vi "SERIAL_StreamProcessor.vi"() -> ()   [LabVIEW 2014, in "navX-MXP IMU.lvlib"]
uses:
  navX-MXP IMU.lvlib
  COMMON/TypeDefs/navX Device TypeDef.ctl
  COMMON/TypeDefs/Value TypeDefs/navX Interface Protocol.ctl
  <vilib>/Rock Robotics/WPI/SPI/WPI_SPIDevRef.ctl
  <vilib>/Rock Robotics/SystemInterfaces/Typedef/FPGA_TypedefDigitalModule.ctl
  <vilib>/Rock Robotics/SystemInterfaces/spilib/spi_bus.ctl
  <vilib>/Rock Robotics/WPI/I2C/WPI_I2CDevRef.ctl
  <vilib>/Rock Robotics/SystemInterfaces/i2clib/i2c_bus.ctl
  <vilib>/Rock Robotics/WPI/SerialPort/WPI_SerialPortRef.ctl
  COMMON/TypeDefs/Data TypeDefs/navX Board Information.ctl
  COMMON/TypeDefs/Value TypeDefs/navX NAVX_BOARD_CAPABILITY.ctl
  COMMON/TypeDefs/Value TypeDefs/navX NAVX_BOARD_YAW_AXIS.ctl
  COMMON/TypeDefs/Data TypeDefs/navX Status Data.ctl
  COMMON/TypeDefs/Value TypeDefs/navX NAVX_OP_STATUS.ctl
  COMMON/TypeDefs/Value TypeDefs/navX NAVX_CAL_STATUS.ctl
  COMMON/TypeDefs/Value TypeDefs/navX NAVX_SELFTEST_STATUS.ctl
  COMMON/TypeDefs/Value TypeDefs/navX NAVX_SENSOR_STATUS.ctl
  COMMON/TypeDefs/Data TypeDefs/navX Offsets Data.ctl
  COMMON/TypeDefs/Value TypeDefs/navX Update Rate.ctl
  COMMON/TypeDefs/Value TypeDefs/navX Serial Mode.ctl
  <vilib>/Platform/TimedLoop/XDataNode/timing_clust.ctl
  <vilib>/Platform/TimedLoop/XDataNode/nitl_modes.ctl
  <vilib>/Platform/TimedLoop/XDataNode/wakeup.ctl
  COMMON/TypeDefs/Value TypeDefs/navX Device Registers.ctl
  <vilib>/Rock Robotics/SystemInterfaces/Utilities/FPGA_UtilitiesRead LocalTime.vi
  <vilib>/platform/TimedLoop/XDataNode/XDataNode.xnode
  <vilib>/Platform/TimedLoop/XDataNode/XDNodeRunTimeDep.lvlib
  NI WPI/NI WPI Serial USB.lvlib
panel:
  in  "navX DevRef":T1={"navX Interface Protocol"=enum."SPI", "navX Interface Protocol TypeDefs"={"SPIDevRef"={"DevStatus"={"status"=FALSE, "code"=0, "source"=""}, "Handle"=0, "Controller"=enum."Controller 1", "SPI Bus"=enum."SPI On-Board, CS0"}, "I2CDevRef"={"DevStatus"={"status"=FALSE, "code"=0, "source"=""}, "Controller"=enum."Controller 1", "Device Address"=0, "Handle"=0, "I2C Bus"=enum."Invalid"}, "SerialPortRef"={"DevStatus"={"status"=FALSE, "code"=0, "source"=""}, "Serial Port Name"=""}}, "navX System Information"={"Board Information"={"WhoAmI (50 | 0x32)"=0, "Board Revision"=0, "Firmware Major Version"=0, "Firmware Minor Version"=0, "NAVX_BOARD_CAPABILITY"={"OMNIMOUNT"=FALSE, "YAW_RESET"=FALSE, "VEL_AND_DISP"=FALSE}, "NAVX_BOARD_YAW_AXIS"={"BOARD_YAW_AXIS_UP"=FALSE, "BOARD_YAW_AXIS"=0}}, "Status"={"Update Rate Hz"=0, "Accelerometer Full-Scale Range"=0, "Gyro Full-Scale Range"=0, "NAVX_OP_STATUS"=0, "NAVX_CAL_STATUS"=0, "NAVX_SELFTEST_STATUS"=0, "NAVX_SENSOR_STATUS"={"MOVING"=FALSE, "YAW_STABLE"=FALSE, "MAG_DISTURBANCE"=FALSE, "ALTITUDE_VALID"=FALSE, "SEALEVEL_PRESS_SET"=FALSE, "FUSED_HEADING_VALID"=FALSE}}, "Offsets"={"Yaw"=0.0, "Quat W"=0.0, "Quat X"=0.0, "Quat Y"=0.0, "Quat Z"=0.0}, "LastSampleTimestamp"=0.0, "LastSampleValid"=FALSE}, "navX Common Information"={"Update Rate (4Hz-60Hz)"=50, "refnum name"="", "error"={"status"=FALSE, "code"=0, "source"=""}, "LastFPGATimestamp"=0.0, "Reboot Detected"=FALSE}, "Serial Protocol Extra"={"Loop VI Refnum"=refnum, "Nav6Mode (YPR)"=enum."Raw"}} {"navX Common Information"."Update Rate (4Hz-60Hz)" min=4 max=60 step=1; "navX System Information"."Status"."NAVX_OP_STATUS" items=["INITIALIZING", "SELFTEST_IN_PROGRESS", "ERROR", "IMU_AUTOCAL_IN_PROGRESS", "NORMAL"]; "navX System Information"."Status"."NAVX_CAL_STATUS" items=["IMU_CAL_STATE_MASK"=3, "IMU_CAL_INPROGRESS"=0, "IMU_CAL_ACCUMULATE"=1, "IMU_CAL_COMPLETE"=2, "MAG_CAL_COMPLETE"=4, "BARO_CAL_COMPLETE"=8]; "navX System Information"."Status"."NAVX_SELFTEST_STATUS" items=["COMPLETE"=80, "GYRO_PASSED"=1, "ACCEL_PASSED"=2, "MAG_PASSED"=4, "BARO_PASSED"=8]; "navX Interface Protocol TypeDefs"."I2CDevRef"."Device Address" format="%.0x"}
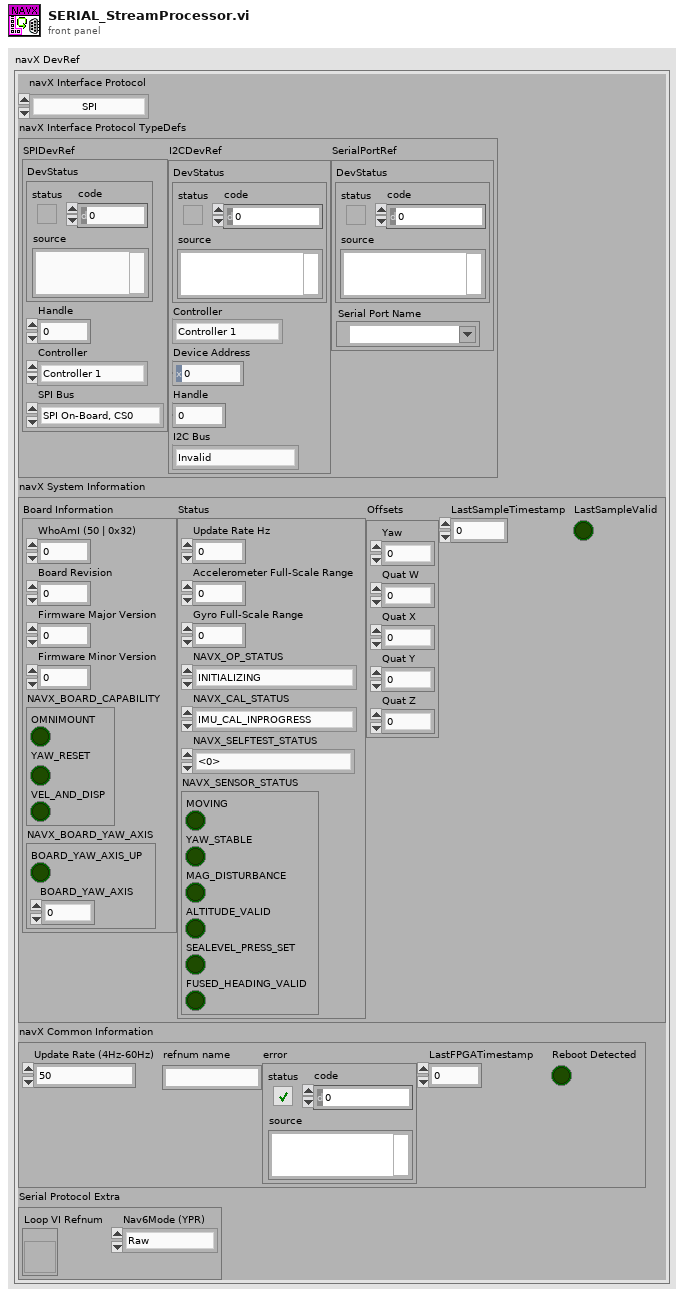
[diagram p1: front panel]
types:
  T1 = typedef "navX-MXP IMU.lvlib/navX Device TypeDef.ctl" = cluster{"navX Interface Protocol":T2, "navX Interface Protocol TypeDefs":cluster{"SPIDevRef":T3, "I2CDevRef":T6, "SerialPortRef":T8}, "navX System Information":cluster{"Board Information":T9, "Status":T12, "Offsets":T17, "LastSampleTimestamp":dbl, "LastSampleValid":bool}, "navX Common Information":cluster{"Update Rate (4Hz-60Hz)":T18, "refnum name":string, "error":errorcluster, "LastFPGATimestamp":dbl, "Reboot Detected":bool}, "Serial Protocol Extra":cluster{"Loop VI Refnum":refnum<vi>, "Nav6Mode (YPR)":T19}}
  T2 = typedef "navX-MXP IMU.lvlib/navX Interface Protocol.ctl" = enum16{"SPI", "I2C", "SERIAL"}
  T3 = typedef "WPI_SPIDevRef.ctl" = cluster{"DevStatus":errorcluster, "Handle":i32, "Controller":T4, "SPI Bus":T5}
  T4 = typedef "FPGA_TypedefDigitalModule.ctl" = enum16{"Controller 1"}
  T5 = typedef "spi_bus.ctl" = enum16{"SPI On-Board, CS0", "SPI On-Board, CS1", "SPI On-Board, CS2", "SPI On-Board, CS3", "SPI MXP", "Invalid"}
  T6 = typedef "WPI_I2CDevRef.ctl" = cluster{"DevStatus":errorcluster, "Controller":T4, "Device Address":u8, "Handle":i32, "I2C Bus":T7}
  T7 = typedef "i2c_bus.ctl" = enum16{"I2C On-Board", "I2C MXP", "Invalid"}
  T8 = typedef "WPI_SerialPortRef.ctl" = cluster{"DevStatus":errorcluster, "Serial Port Name":refnum<visa-resource-name>}
  T9 = typedef "navX-MXP IMU.lvlib/navX Board Information.ctl" = cluster{"WhoAmI (50 | 0x32)":u8, "Board Revision":u8, "Firmware Major Version":u8, "Firmware Minor Version":u8, "NAVX_BOARD_CAPABILITY":T10, "NAVX_BOARD_YAW_AXIS":T11}
  T10 = typedef "navX-MXP IMU.lvlib/navX NAVX_BOARD_CAPABILITY.ctl" = cluster{"OMNIMOUNT":bool, "YAW_RESET":bool, "VEL_AND_DISP":bool}
  T11 = typedef "navX-MXP IMU.lvlib/navX NAVX_BOARD_YAW_AXIS.ctl" = cluster{"BOARD_YAW_AXIS_UP":bool, "BOARD_YAW_AXIS":u8}
  T12 = typedef "navX-MXP IMU.lvlib/navX Status Data.ctl" = cluster{"Update Rate Hz":u8, "Accelerometer Full-Scale Range":u8, "Gyro Full-Scale Range":u16, "NAVX_OP_STATUS":T13, "NAVX_CAL_STATUS":T14, "NAVX_SELFTEST_STATUS":T15, "NAVX_SENSOR_STATUS":T16}
  T13 = typedef "navX-MXP IMU.lvlib/navX NAVX_OP_STATUS.ctl" = u8
  T14 = typedef "navX-MXP IMU.lvlib/navX NAVX_CAL_STATUS.ctl" = u8
  T15 = typedef "navX-MXP IMU.lvlib/navX NAVX_SELFTEST_STATUS.ctl" = u8
  T16 = typedef "navX-MXP IMU.lvlib/navX NAVX_SENSOR_STATUS.ctl" = cluster{"MOVING":bool, "YAW_STABLE":bool, "MAG_DISTURBANCE":bool, "ALTITUDE_VALID":bool, "SEALEVEL_PRESS_SET":bool, "FUSED_HEADING_VALID":bool}
  T17 = typedef "navX-MXP IMU.lvlib/navX Offsets Data.ctl" = cluster{"Yaw":dbl, "Quat W":dbl, "Quat X":dbl, "Quat Y":dbl, "Quat Z":dbl}
  T18 = typedef "navX-MXP IMU.lvlib/navX Update Rate.ctl" = u8
  T19 = typedef "navX-MXP IMU.lvlib/navX Serial Mode.ctl" = enum16{"Raw", "Processed"}
  T20 = typedef "XDNodeRunTimeDep.lvlib/timing_clust.ctl" = cluster{"Expected End [f-1]":u64, "Actual End [f-1]":u64, "Finished Late? [f-1]":bool, "Expected End [i-1]":u64, "Actual End [i-1]":u64, "Finished Late? [i-1]":bool, "Expected Start [i]":u64, "Actual Start [i]":u64, "Expected Start [f]":u64, "Actual Start [f]":u64, "Source Name":string, "Structure Name":string, "Period":i64, "Deadline":i64, "Offset":i64, "Start":i64, "Priority":i32, "Timeout":i32, "Mode":T21, "Wakeup Reason":T22, "Error":errorcluster, "Source Type":string, "Secondary Source Type":string, "Global End Time":u64, "Global Start Time":u64, "Frame Duration":u64, "Iteration Duration":u64, "Assigned CPU":i32, "I/O Scan Engine Mode":u32}
  T21 = typedef "XDNodeRunTimeDep.lvlib/nitl_modes.ctl" = enum32{"No Change", "Process missed periods, maintain original phase", "Discard missed periods, maintain original phase", "Process missed periods, ignore original phase", "Discard missed periods, ignore original phase"}
  T22 = typedef "XDNodeRunTimeDep.lvlib/wakeup.ctl" = enum32{"Normal", "Aborted", "Asynchronous wakeup", "Timing source error", "Timed loop error", "Timeout"}
  T23 = typedef "navX-MXP IMU.lvlib/navX Device Registers.ctl" = u8
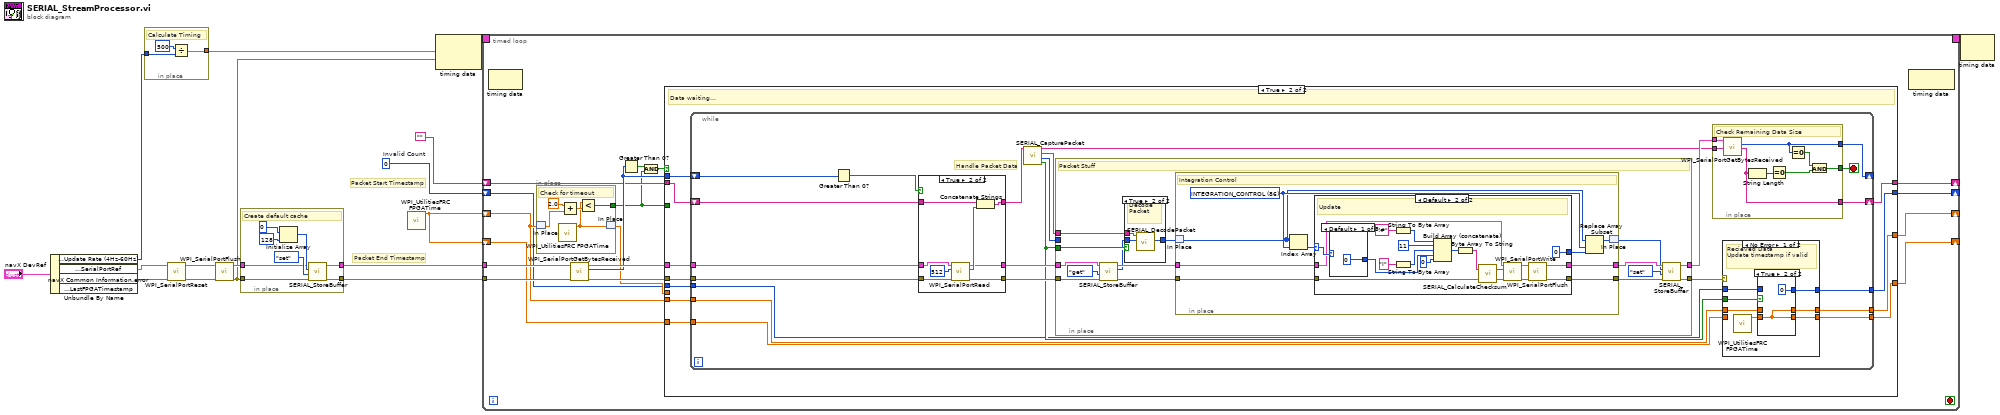
[diagram p0: block diagram]
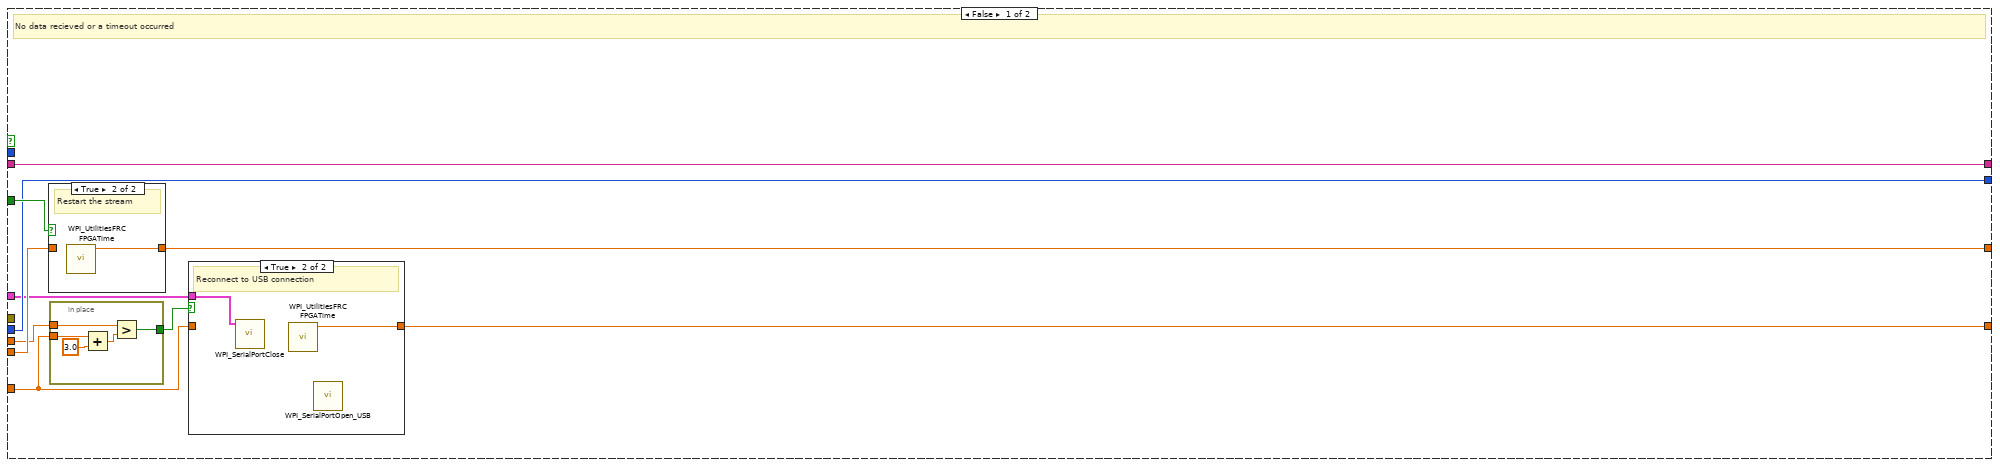
[diagram p2: hidden frame]
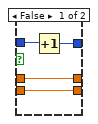
[diagram p5: hidden frame]
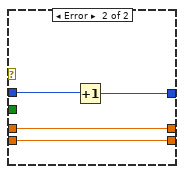
[diagram p6: hidden frame]
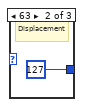
[diagram p9: hidden frame]
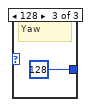
[diagram p10: hidden frame]
diagram:
  w1 = 0  # Invalid Count
  # "Packet End Timestamp"
  # "Packet Start Timestamp"
  n1 = Unbundle By Name("navX DevRef") -> ("navX Common Information.Update Rate (4Hz-60Hz)"=w6:T18, "navX Interface Protocol TypeDefs.SerialPortRef"=w9:T8, "navX Common Information.error"=w8:errorcluster)  [unwired: 1 out]
  n2 = in-place {
    in-place-border: w6 -> [w18]
    in-place-border: [w17] -> w7
    # "Calculate Timing"
    n3 = Divide(x=500, y=w18) -> (x/y=w17:dbl)
  }
  n4 = call <vilib>:"WPI_SerialPortReset.vi"("error in (no error)"=w8, "SerialPortRef"=w9) -> ("error out"=w14:errorcluster, "SerialPortRef"=w13:T8)  [unwired: 8 in]
  n5 = call <vilib>:"WPI_SerialPortFlush.vi"("error in (no error)"=w14, "SerialPortRef"=w13) -> ("error out"=w4:errorcluster, "SerialPortRef"=w5:T8)  [unwired: 8 in]
  n6 = in-place {
    in-place-border: w5 -> [w23]
    in-place-border: w4 -> [w22]
    in-place-border: [w21] -> w3
    in-place-border: [w20] -> w2
    # "Create default cache"
    n7 = Initialize Array(u8 0 ("Received Data"), u8 128 ("hex")) -> (w24:u8[])
    n8 = call "SERIAL_StoreBuffer.vi"("error in (no error)"=w22, "Access Type"=enum16{"set", "get", "delete"}."set", "navX Data"=w24, "SerialPortRef"=w23) -> ("error out"=w21:errorcluster, "SerialPortRef"=w20:T8)  [unwired: 5 in, 1 out]
  }
  n9 = call <vilib>:"WPI_UtilitiesFRC FPGATime.vi"() -> ("FPGA Time"=w12:dbl)  [unwired: 10 in, 1 out]
  n10 = node-c288(w7, w4) -> (w16:T20)
  n11 = timed-loop {
    timing: w16 -> [_]
    timing-out: [_] -> w15
    tunnel: w2 -> [w39]
    tunnel: w3 -> [w44]
    shift-right: [w36] -> _
    shift-left: w12 -> [w31]
    shift-right: [w35] -> _
    shift-left: w12 -> [w34]
    shift-right: [w32] -> _
    shift-left: "" -> [w37]
    shift-right: [w28] -> _
    shift-left: w1 -> [w29]
    stop <- _ stop-if-true
    n12 = node-c288() -> ()  [unwired: 1 in, 1 out]
    n13 = in-place {
      in-place-border: [w189] -> w33
      # "Check for timeout"
      n14 = in-place-match #1(w31) -> (w188:dbl)
      n15 = call <vilib>:"WPI_UtilitiesFRC FPGATime.vi"() -> ("FPGA Time"=w187:dbl)  [unwired: 10 in, 1 out]
      n16 = Add(x=2.0, y=w188) -> (x+y=w190:dbl)
      n17 = Less?(x=w187, y=w190) -> (x < y?=w189:bool)
      n18 = in-place-match #1(w187) -> (w30:dbl)
    }
    n19 = call <vilib>:"WPI_SerialPortGetBytesReceived.vi"("error in (no error)"=w44, "SerialPortRef"=w39) -> ("error out"=w40:errorcluster, "Bytes at Port"=w38:u32, "SerialPortRef"=w41:T8)  [unwired: 7 in]
    n20 = Greater Than 0?(x=w38) -> (x > 0?=w43:bool)
    n21 = Compound Arithmetic op=AND(w43, w33) -> (w42:bool)
    n22 = case shown="True" w42 {
      tunnel: w41 -> [w45 w74]
      tunnel: w40 -> [_ w73]
      tunnel: w38 -> [_ w75]
      tunnel: w37 -> [w47 w72]
      tunnel: w31 -> [w53 w71]
      tunnel: [w48 w70] -> w36
      tunnel: [w49 w69] -> w35
      tunnel: w34 -> [w50 w68]
      tunnel: w33 -> [w54 _]
      tunnel: w30 -> [w52 _]
      tunnel: [w47 w67] -> w32
      tunnel: w29 -> [w46 w66]
      tunnel: [w46 w65] -> w28
      frame False {
        # "No data recieved or a timeout occurred"
        n23 = case shown="True" w54 {
          tunnel: [w63 w64] -> w48
          tunnel: w53 -> [w63 _]
          frame False {
          }
          frame True {
            # "Restart the stream"
            n24 = call <vilib>:"WPI_UtilitiesFRC FPGATime.vi"() -> ("FPGA Time"=w64:dbl)  [unwired: 10 in, 1 out]
          }
        }
        n25 = in-place {
          in-place-border: w52 -> [w57]
          in-place-border: [w56] -> w51
          in-place-border: w50 -> [w55]
          n26 = Add(x=w55, y=3.0) -> (x+y=w58:dbl)
          n27 = Greater?(x=w57, y=w58) -> (0:w56:bool)
        }
        n28 = case shown="True" w51 {
          tunnel: [w60 w62] -> w49
          tunnel: w50 -> [w60 _]
          tunnel: w45 -> [_ w61]
          frame False {
          }
          frame True {
            # "Reconnect to USB connection"
            n29 = call <vilib>:"WPI_SerialPortClose.vi"("SerialPortRef"=w61) -> ()  [unwired: 10 in, 1 out]
            n30 = call <vilib>:"WPI_UtilitiesFRC FPGATime.vi"() -> ("FPGA Time"=w62:dbl)  [unwired: 10 in, 1 out]
            n31 = call "WPI_SerialPortOpen_USB.vi"() -> ()  [unwired: 14 in, 2 out]
          }
        }
      }
      frame True {
        # "Data waiting..."
        n32 = while {
          shift-right: [w82] -> _
          shift-left: w75 -> [w98]
          tunnel: w74 -> [w96]
          tunnel: w73 -> [w95]
          shift-right: [w79] -> w67
          shift-left: w72 -> [w94]
          tunnel: w71 -> [w88]
          tunnel: [w87] -> w70
          tunnel: [w86] -> w69
          tunnel: w68 -> [w85]
          tunnel: w66 -> [w77]
          tunnel: [w76] -> w65
          stop <- w81 stop-if-true
          # "Handle Packet Data"
          n33 = Greater Than 0?(x=w98) -> (x > 0?=w97:bool)
          n34 = case shown="True" w97 {
            tunnel: w96 -> [w176 w185]
            tunnel: w95 -> [w177 w184]
            tunnel: w94 -> [w178 w182]
            tunnel: [w178 w181] -> w93
            tunnel: [w177 w180] -> w89
            tunnel: [w176 w179] -> w90
            frame False {
            }
            frame True {
              n35 = call <vilib>:"WPI_SerialPortRead.vi"("error in (no error)"=w184, "Num Bytes to Read"=u32 512, "SerialPortRef"=w185) -> ("error out"=w180:errorcluster, "Buffer"=w183:string, "SerialPortRef"=w179:T8)  [unwired: 6 in]
              n36 = Concatenate Strings(w182, w183) -> (w181:string)
            }
          }
          n37 = call "SERIAL_CapturePacket.vi"("Stream"=w93) -> ("Packet Located"=w78:bool, "Packet Length"=w91:i32, "Packet"=w92:string, "Stream"=w80:string)  [unwired: 7 in]
          n38 = in-place {
            in-place-border: w92 -> [w126]
            in-place-border: w91 -> [_]
            in-place-border: w78 -> [w127]
            in-place-border: w90 -> [w137]
            in-place-border: w89 -> [w134]
            in-place-border: [w133] -> w84
            in-place-border: [w128] -> w83
            # "Packet Stuff"
            n39 = call "SERIAL_StoreBuffer.vi"("error in (no error)"=w134, "Access Type"=enum16{"set", "get", "delete"}."get", "SerialPortRef"=w137) -> ("error out"=w132:errorcluster, "navX Data"=w125:u8[], "SerialPortRef"=w130:T8)  [unwired: 6 in]
            n40 = case shown="True" w127 {
              tunnel: w126 -> [_ w141]
              tunnel: w125 -> [w138 w140]
              tunnel: [w138 w139] -> w124
              frame False {
              }
              frame True {
                # "Decode Packet"
                n41 = call "SERIAL_DecodePacket.vi"("Data"=w140, "Packet"=w141) -> ("Data"=w139:u8[])  [unwired: 8 in, 1 out]
              }
            }
            n42 = in-place {
              in-place-border: [w147] -> w129
              in-place-border: w130 -> [w146]
              in-place-border: w132 -> [w145]
              in-place-border: [w144] -> w131
              w149 = T23 86 items=["WHOAMI"=0, "HW_REV"=1, "FW_VER_MAJOR"=2, "FW_VER_MINOR"=3, "UPDATE_RATE_HZ"=4, "ACCEL_FSR_G"=5, "GYRO_FSR_DPS"=6, "OP_STATUS"=8, "CAL_STATUS"=9, "SELFTEST_STATUS"=10, "CAPABILITY_FLAGS_L"=11, "CAPABILITY_FLAGS_H"=12, "SENSOR_STATUS"=16, "TIMESTAMP"=18, "YAW"=22, "PITCH"=24, "ROLL"=26, "HEADING"=28, "FUSED_HEADING"=30, "ALTITUDE_I"=32, "ALTITUDE_D"=34, "LINERA_ACC_X"=36, "LINERA_ACC_Y"=38, "LINERA_ACC_Z"=40, "QUAT_W"=42, "QUAT_X"=44, "QUAT_Y"=46, "QUAT_Z"=48, "MPU_TEMP_C"=50, "GYRO_X"=52, "GYRO_Y"=54, "GYRO_Z"=56, "ACC_X"=58, "ACC_Y"=60, "ACC_Z"=62, "MAG_X"=64, "MAG_Y"=66, "MAG_Z"=68, "PRESSURE_I"=70, "PRESSURE_D"=72, "PRESSURE_TEMP"=74, "YAW_OFFSET"=76, "QUAT_OFFSET_W"=78, "QUAT_OFFSET_X"=80, "QUAT_OFFSET_Y"=82, "QUAT_OFFSET_Z"=84, "INTEGRATION_CONTROL"=86, "VELOCITY_X"=88, "VELOCITY_Y"=92, "VELOCITY_Z"=96, "DISPLACMENT_X"=100, "DISPLACMENT_Y"=104, "DISPLACEMENT_Z"=108] ("Device Register")
              # "Integration Control"
              n43 = in-place-match #2(w124) -> (w143:u8[])
              n44 = Index Array(array=w143, index=w149) -> (element=w150:u8)
              n45 = case shown="Default" w150 {
                selector: w150 -> [w153 w171]
                tunnel: [w153 0] -> w148
                tunnel: [w152 w157] -> w147
                tunnel: [w151 w156] -> w144
                tunnel: w146 -> [w152 w155]
                tunnel: w145 -> [w151 w154]
                frame 0 {
                }
                frame Default {
                  # "Update"
                  n46 = case shown="Default" w171 {
                    tunnel: [u8 0 u8 127 u8 128] -> w164
                    frame Default {
                    }
                    frame 63 {
                      # "Displacement"
                    }
                    frame 128 {
                      # "Yaw"
                    }
                  }
                  n47 = String To Byte Array(string="!#") -> (unsigned byte array=w168:u8[])
                  n48 = String To Byte Array(string="I" ("format string")) -> (unsigned byte array=w166:u8[])
                  n49 = Build Array (concatenate)(w168, u8 11, w166, w164, u8 0) -> (w163:u8[])
                  n50 = Byte Array To String(unsigned byte array=w163) -> (string=w162:string)
                  n51 = call "SERIAL_CalculateChecksum.vi"("error in"=w154, "Content"=w162) -> ("error out"=w158:errorcluster, "Teminated Content"=w159:string)
                  n52 = call <vilib>:"WPI_SerialPortWrite.vi"("error in (no error)"=w158, "Buffer"=w159, "SerialPortRef"=w155) -> ("error out"=w161:errorcluster, "SerialPortRef"=w160:T8)  [unwired: 6 in, 1 out]
                  n53 = call <vilib>:"WPI_SerialPortFlush.vi"("error in (no error)"=w161, "SerialPortRef"=w160) -> ("error out"=w156:errorcluster, "SerialPortRef"=w157:T8)  [unwired: 8 in]
                }
              }
              n54 = Replace Array Subset(array=w143, new element=w148, index=w149) -> (w142:u8[])
              n55 = in-place-match #2(w142) -> (w123:u8[])
            }
            n56 = call "SERIAL_StoreBuffer.vi"("error in (no error)"=w131, "Access Type"=enum16{"set", "get", "delete"}."set", "navX Data"=w123, "SerialPortRef"=w129) -> ("error out"=w133:errorcluster, "SerialPortRef"=w128:T8)  [unwired: 5 in, 1 out]
          }
          n57 = in-place {
            in-place-border: w83 -> [w105]
            in-place-border: [w104] -> w82
            in-place-border: [w99] -> w79
            in-place-border: [w101] -> w81
            in-place-border: w80 -> [w99]
            # "Check Remaining Data Size"
            n58 = call <vilib>:"WPI_SerialPortGetBytesReceived.vi"("SerialPortRef"=w105) -> ("Bytes at Port"=w104:u32)  [unwired: 8 in, 2 out]
            n59 = String Length(string=w99) -> (length=w103:i32)
            n60 = Equal To 0?(x=w103) -> (x = 0?=w100:bool)
            n61 = Equal To 0?(x=w104) -> (x = 0?=w102:bool)
            n62 = Compound Arithmetic op=AND(w102, w100) -> (w101:bool)
          }
          n63 = case shown="No Error" w84 {
            tunnel: [w112 w122] -> w87
            tunnel: w88 -> [w111 w122]
            tunnel: w85 -> [_ w121]
            tunnel: [w110 w121] -> w86
            tunnel: w78 -> [w108 _]
            tunnel: w77 -> [w107 w120]
            tunnel: [w106 w119] -> w76
            frame No Error {
              # "Recieved Data\nUpdate timestamp if valid"
              n64 = call <vilib>:"WPI_UtilitiesFRC FPGATime.vi"() -> ("FPGA Time"=w109:dbl)  [unwired: 10 in, 1 out]
              n65 = case shown="True" w108 {
                tunnel: [w116 w118] -> w112
                tunnel: w111 -> [w116 _]
                tunnel: [w115 w118] -> w110
                tunnel: w109 -> [w115 w118]
                tunnel: w107 -> [w114 _]
                tunnel: [w113 0] -> w106
                frame False {
                  n66 = Increment(x=w114) -> (x+1=w113:i32)
                }
                frame True {
                }
              }
            }
            frame Error {
              n67 = Increment(x=w120) -> (x+1=w119:i32)
            }
          }
        }
      }
    }
    n68 = node-c288() -> ()  [unwired: 1 in, 1 out]
  }
  n69 = node-c288(w15) -> ()  [unwired: 1 out]
